vi "Data Changed.vi"(1 "Data":variant) -> (0 "Changed?":bool=TRUE)   [LabVIEW 2011]
doc: "Returns true if input data has changed.\nFirst call returns true.\n\n\nVersion 1.0 - 02/27/2013\n\nPhaeron, Inc.\nwww.phaeron.com\ninfo@phaeron.com"
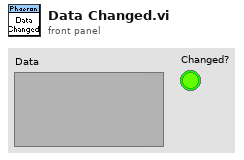
[diagram p1: front panel]
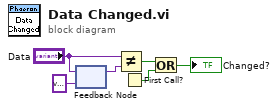
[diagram p0: block diagram]
diagram:
  n1 = feedback-in #1("Data") -> ()
  n2 = feedback #1(variant ("Data")) -> (w5:variant)
  n3 = Not Equal?(x="Data", y=w5) -> (x != y?=w3:bool)
  n4 = First Call?() -> (First Call?: T/F=w1:bool)
  n5 = Or(x=w3, y=w1) -> (x .or. y?=→"Changed?":bool)
